vi "TC calibrate.vi"(10 "TC in":dbl[](array[numeric])) -> (2 "TC out":sgl[](array[numeric]))   [LabVIEW 2014]
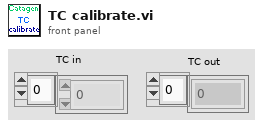
[diagram p1: front panel]
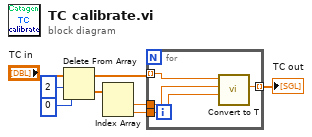
[diagram p0: block diagram]
diagram:
  n1 = Delete From Array(array="TC in", length=2, index=0) -> (deleted portion=w4:dbl[], array with subset deleted=w5:dbl[])
  n2 = Index Array(array=w4) -> (element #1=w3:dbl, element #2=w2:dbl)  [unwired: 2 in]
  n3 = for {
    tunnel: w2 -> [w11]
    tunnel: w3 -> [w12]
    tunnel: w5 -> [w10] mode=indexing
    tunnel: [w9] -> w1 mode=indexing
    n4 = call "Convert to T.vi"("CJC"=w11, "AutoZero"=w12, "TC Input"=w10) -> ("Linearized Temperature"=w9:sgl)  [unwired: 8 in]
  }
  "TC out" <- w1
